vi "Get Message Endpoint.vi"(8 "error in":errorcluster, 11 "message in":T1 format="%.0x") -> (0 "error out":errorcluster, 2 "message endpoint":T2, 3 "message out":T1 format="%.0x")   [LabVIEW 2020, in "AIM MIL-STD-1553 Scripting.lvlib"]
uses:
  AIM MIL-STD-1553 Scripting.lvlib
  <vilib>/NI VeriStand/Custom Device API/Custom Device Item Ref.ctl
  Shared/Terminal Endpoint.ctl
  Shared/Address.ctl
  <vilib>/NI VeriStand/Custom Device API/Custom Device API.lvlib
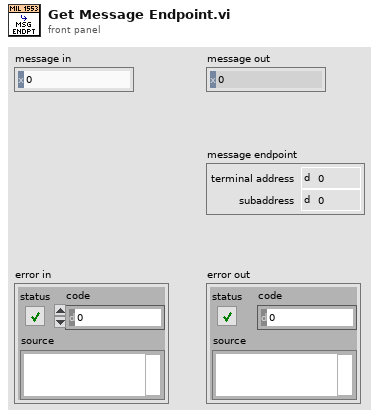
[diagram p1: front panel]
types:
  T1 = typedef "Custom Device API.lvlib/Custom Device Item Ref.ctl" = u64
  T2 = typedef "Terminal Endpoint.ctl" = cluster{"terminal address":T3, "subaddress":T3}
  T3 = typedef "Address.ctl" = u16
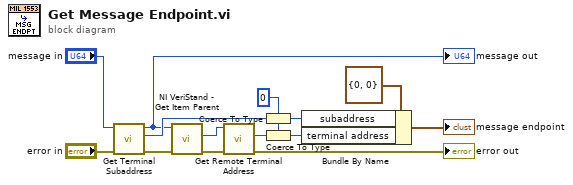
[diagram p0: block diagram]
diagram:
  w3 = T3 0 ("subaddress")
  n1 = call "Get Terminal Subaddress.vi"("error in"="error in", "subaddress in"="message in") -> ("error out"=w11:errorcluster, "subaddress value"=w7:T3, "subaddress out"=w1:T1)  [unwired: 6 in, 1 out]
  "message out" <- w1
  n2 = call <vilib>:"NI VeriStand - Get Item Parent.vi"("error in (no error)"=w11, "Item Ref in"=w1) -> ("error out"=w9:errorcluster, "Parent Ref"=w10:T1)  [unwired: 6 in, 2 out]
  n3 = call "Get Remote Terminal Address.vi"("error in"=w9, "remote terminal"=w10) -> ("error out"=→"error out":errorcluster, "terminal address"=w5:T3)  [unwired: 6 in, 2 out]
  n4 = Coerce To Type(0:w7, 1:w3) -> (2:w6:T3)
  n5 = Coerce To Type(0:w5, 1:w3) -> (2:w4:T3)
  n6 = Bundle By Name(cluster=T2 {"terminal address"=0, "subaddress"=0} ("endpoint Rx"), "subaddress"=w6, "terminal address"=w4) -> (→"message endpoint":T2)
